vi "BasicTrig.vi"(8 "error in (no error)":errorcluster, 11 "reference":refnum<k24>) -> (0 "error out":errorcluster, 1 "PretriggerCount":i32, 2 "Edge":i32(ring) items=["Rising", "Falling"], 3 "reference out":refnum<k24>, 4 "Type":i32(ring) items=["None", "AnalogEdge", "DigitalLevel", "DigitalEdge"], 5 "Slope":i32(ring) items=["Rising", "Falling"], 6 "DigitalLevel":i32(ring) items=["High", "Low"], 7 "AnalogLevel":dbl)   [LabVIEW 2009]
uses:
  C:/Program Files/National Instruments/LabVIEW 2009/vi.lib/ULx/ULx_LV.dll
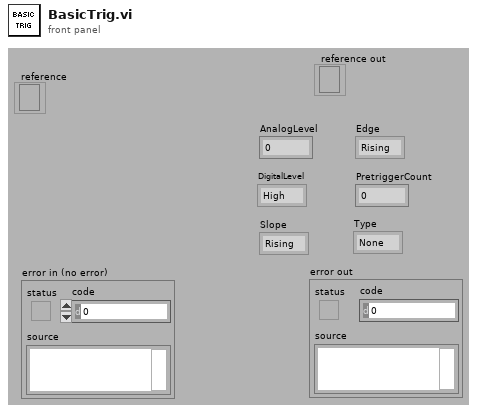
[diagram p1: front panel]
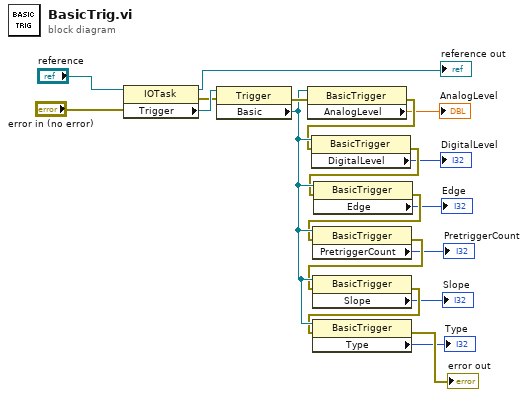
[diagram p0: block diagram]
diagram:
  n1 = property class="IOTask"(reference="reference", error in="error in (no error)") -> (reference out=→"reference out":refnum<k24>, error out=w18:errorcluster, "Trigger"=w19:refnum<k24>)
  n2 = property class="Trigger"(reference=w19, error in=w18) -> (error out=w17:errorcluster, "Basic"=w16:refnum<k24>)  [unwired: 1 out]
  n3 = property class="BasicTrigger"(reference=w16, error in=w17) -> (error out=w15:errorcluster, "AnalogLevel"=→"AnalogLevel":dbl)  [unwired: 1 out]
  n4 = property class="BasicTrigger"(reference=w16, error in=w15) -> (error out=w14:errorcluster, "DigitalLevel"=→"DigitalLevel":i32)  [unwired: 1 out]
  n5 = property class="BasicTrigger"(reference=w16, error in=w14) -> (error out=w13:errorcluster, "Edge"=→"Edge":i32)  [unwired: 1 out]
  n6 = property class="BasicTrigger"(reference=w16, error in=w13) -> (error out=w12:errorcluster, "PretriggerCount"=→"PretriggerCount":i32)  [unwired: 1 out]
  n7 = property class="BasicTrigger"(reference=w16, error in=w12) -> (error out=w11:errorcluster, "Slope"=→"Slope":i32)  [unwired: 1 out]
  n8 = property class="BasicTrigger"(reference=w16, error in=w11) -> (error out=→"error out":errorcluster, "Type"=→"Type":i32)  [unwired: 1 out]
